vi "Calc min points to read.vi"(3 "error in":errorcluster, 4 "Target number of points":u64, 5 "Logging queue element":T1={"Imaging Protocol"=enum."Live Imaging", "Number of Trials"=0, "Frame Size"=512, "# Averaged frames"=0, "Dwell time (us)"=0.0, "Index of Z-plane"=0, "Timelapse?"=FALSE, "Logging process is active"=FALSE, "Speed logging enabled"=FALSE, "tdms file ref"=refnum, "path"=path "", "Trial Number"=0, "Expected # points acquired"=FALSE, "Manually stopped"=FALSE, "Last trial"=FALSE, "Ch0 data"=[], "Ch1 data"=[], "Image Time"=[], "Continuous Time"=[], "Points acquired"={"Ch0 last trial"=0, "Ch1 last trial"=0, "All trials"=0}, "HW Timings File"=refnum} {"Frame Size" items=["100X100"=100, "128X128"=128, "200X200"=200, "256X256"=256, "512X512"=512, "1024x1024"=1024, "2048x2048"=2048]; "Dwell time (us)" format="%#.6g"}) -> (0 "error out":errorcluster, 2 "Read at least # points":u32)   [LabVIEW 2017]
uses:
  Typedefs/Logging queue element.ctl
  Typedefs/Imaging Protocols enum.ctl
  Typedefs/Frame Size.ctl
  Typedefs/Acquired points count.ctl
panel:
  in  "Very important value":u64=200000
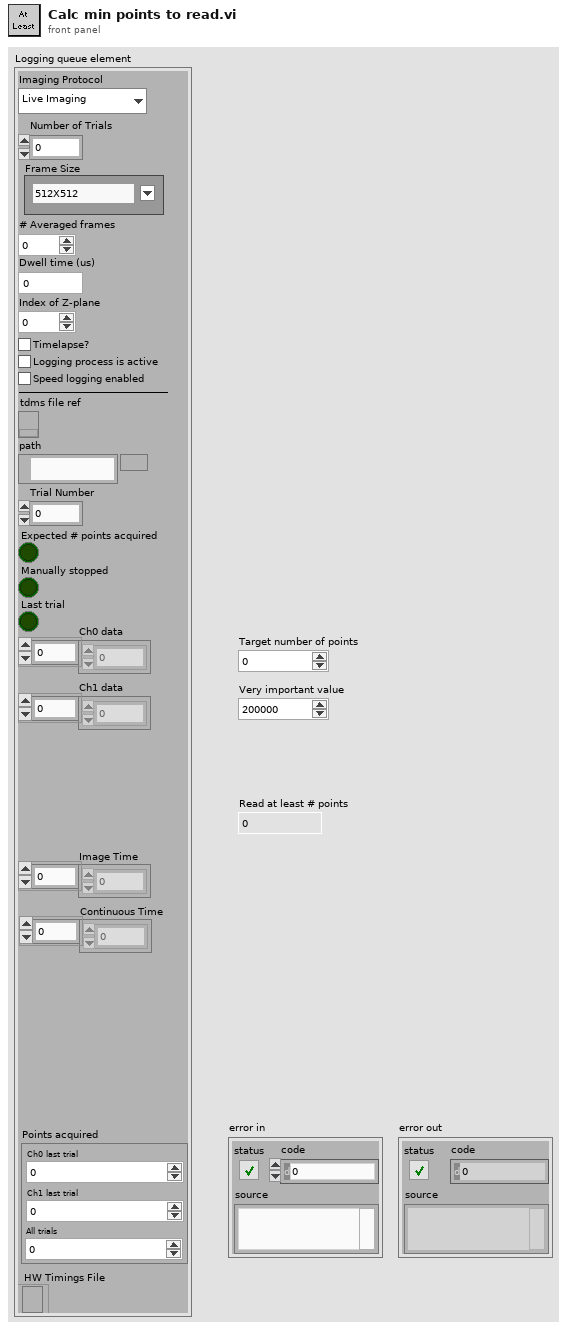
[diagram p1: front panel]
types:
  T1 = typedef "Logging queue element.ctl" = cluster{"Imaging Protocol":T2, "Number of Trials":u16, "Frame Size":T3, "# Averaged frames":u16, "Dwell time (us)":dbl, "Index of Z-plane":i32, "Timelapse?":bool, "Logging process is active":bool, "Speed logging enabled":bool, "tdms file ref":refnum<k34>, "path":path, "Trial Number":i32, "Expected # points acquired":bool, "Manually stopped":bool, "Last trial":bool, "Ch0 data":u32[], "Ch1 data":u32[], "Image Time":u64[], "Continuous Time":u64[], "Points acquired":T4, "HW Timings File":refnum<file>}
  T2 = typedef "Imaging Protocols enum.ctl" = enum16{"AOL Z-Stack", "Motor Z Stack", "Functional Acquisition", "Single Plane Acquisition", "Volume Acquisition", "Live Imaging", "Live Plane Imaging", "Live Volume Imaging"}
  T3 = typedef "Frame Size.ctl" = u16
  T4 = typedef "Acquired points count.ctl" = cluster{"Ch0 last trial":u64, "Ch1 last trial":u64, "All trials":u64}
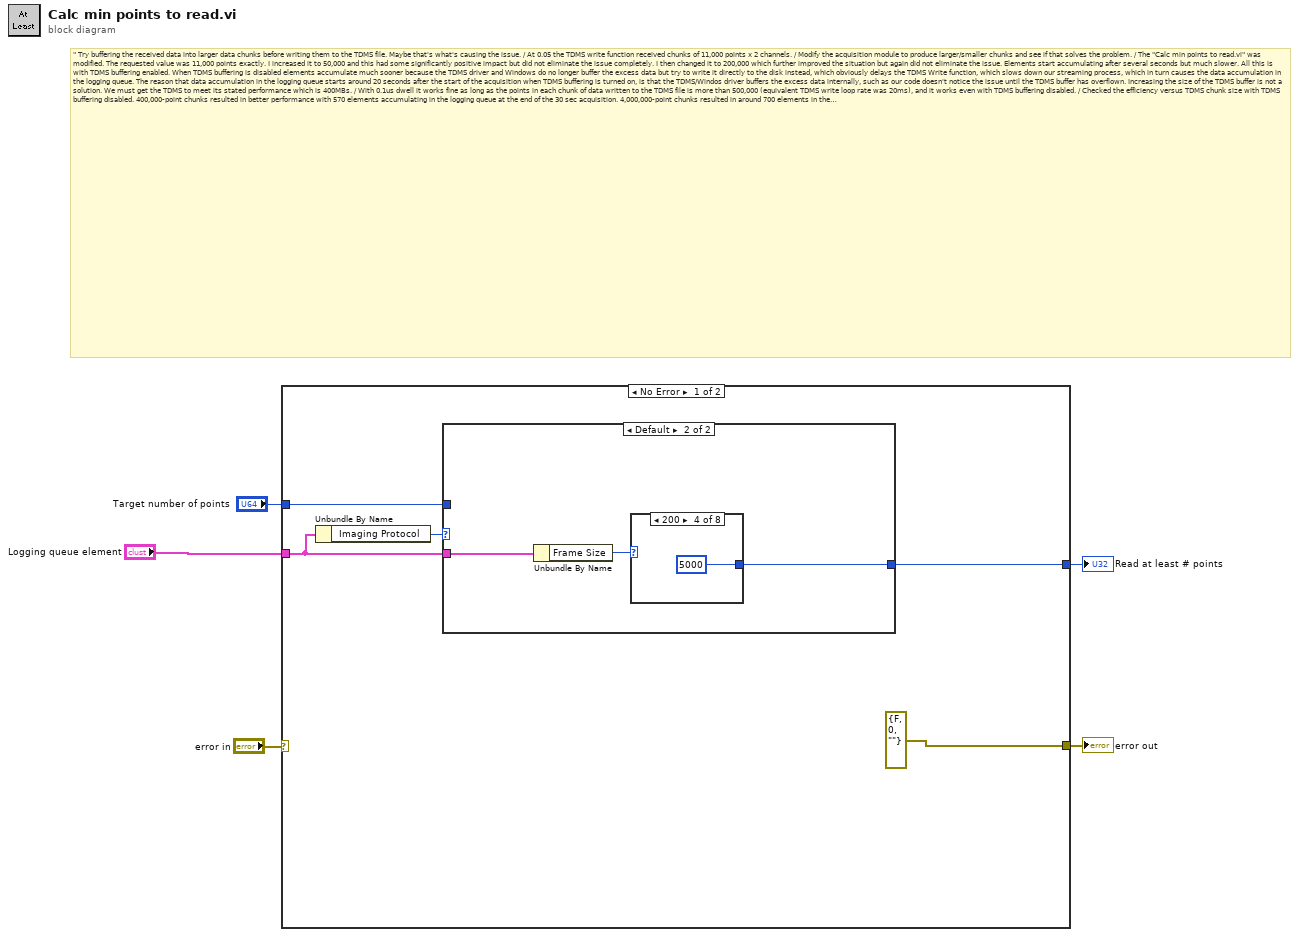
[diagram p0: block diagram]
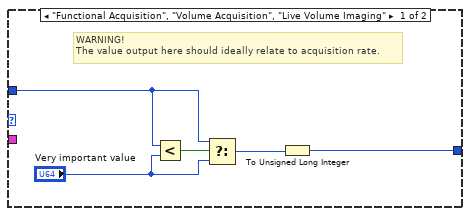
[diagram p2: hidden frame]
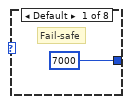
[diagram p3: hidden frame]
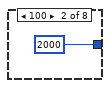
[diagram p4: hidden frame]
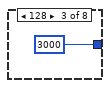
[diagram p5: hidden frame]
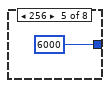
[diagram p6: hidden frame]
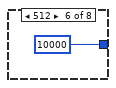
[diagram p7: hidden frame]
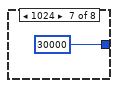
[diagram p8: hidden frame]
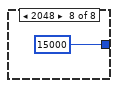
[diagram p9: hidden frame]
diagram:
  # "\"\tTry buffering the received data into larger data chunks before writing them to the TDMS file. Maybe that's what's causing the issue. / At 0.05 the TDMS write function received chunks of 11,000 points x 2 channels. / Modify the acquisition module to produce larger/smaller chunks and see if that solves the problem. / The \"Calc min points to read.vi\" was modified. The requested value was 11,000 points exactly. I increased it to 50,000 and this had some significantly positive impact but did not eliminate the issue completely. I then changed it to 200,000 which further improved the situation but again did not eliminate the issue. Elements start accumulating after several seconds but much slower. All this is with TDMS buffering enabled. When TDMS buffering is disabled elements accumulate much sooner because the TDMS driver and Windows do no longer buffer the excess data but try to write it directly to the disk instead, which obviously delays the TDMS Write function, which slows down our streaming process, which in turn causes the data accumulation in the logging queue. The reason that data accumulation in the logging queue starts around 20 seconds after the start of the acquisition when TDMS buffering is turned on, is that the TDMS/Windos driver buffers the excess data internally, such as our code doesn't notice the issue until the TDMS buffer has overflown. Increasing the size of the TDMS buffer is not a solution. We must get the TDMS to meet its stated performance which is 400MBs. / With 0.1us dwell it works fine as long as the points in each chunk of data written to the TDMS file is more than 500,000 (equivalent TDMS write loop rate was 20ms), and it works even with TDMS buffering disabled. / Checked the efficiency versus TDMS chunk size with TDMS buffering disabled. 400,000-point chunks resulted in better performance with 570 elements accumulating in the logging queue at the end of the 30 sec acquisition. 4,000,000-point chunks resulted in around 700 elements in the queue (note each element contained 4 Million points) as compared to the previous case where each element contained just 400,000 points). With 4,000-point chunks there were over 10,000 points in the queue before an error occurred. With 40,000-point chunks the queue size reached 3500 elements.\n4,000,000 -> 700 ' 2800M points in the queue\n400,000   -> 570 ' 228M points in the queue\n300,000  -> 600 ' 180M points\n200,000   -> 550  ' 110M points\n100,000   -> 2100 ' 210M points\n40,000    -> 3500 ' 140M points\n4,000      -> >10,000 ' N/A\nI set the chunk size to 200,000 points at least for now since it appears to be the most optimal value."
  n1 = case shown="No Error" "error in" {
    selector: "error in" -> [_ w27]
    tunnel: [w10 _] -> w5
    tunnel: "Logging queue element" -> [w6 _]
    tunnel: "Target number of points" -> [w8 _]
    tunnel: [errorcluster {"status"=FALSE, "code"=0, "source"=""} ("error out") w27] -> w3
    frame No Error {
      n2 = Unbundle By Name(w6) -> ("Imaging Protocol"=w9:T2)
      n3 = case shown="Default" w9 {
        tunnel: [w11 w18] -> w10
        tunnel: w6 -> [_ w16]
        tunnel: w8 -> [w14 _]
        frame "Functional Acquisition", "Volume Acquisition", "Live Volume Imaging" {
          # "WARNING!\nThe value output here should ideally relate to acquisition rate."
          n4 = Less?(x=w14, y="Very important value") -> (x < y?=w15:bool)
          n5 = Select(t=w14, s=w15, f="Very important value") -> (s? t:f=w12:u64)
          n6 = To Unsigned Long Integer(number=w12) -> (unsigned 32bit integer=w11:u32)
        }
        frame Default {
          n7 = Unbundle By Name(w16) -> ("Frame Size"=w17:T3)
          n8 = case shown="200" w17 {
            tunnel: [u32 7000 ("unsigned 32bit integer") u32 2000 ("unsigned 32bit integer") u32 3000 ("unsigned 32bit integer") u32 5000 ("unsigned 32bit integer") u32 6000 ("unsigned 32bit integer") u32 10000 ("unsigned 32bit integer") u32 30000 ("unsigned 32bit integer") u32 15000 ("unsigned 32bit integer")] -> w18
            frame Default {
              # "Fail-safe"
            }
            frame 100 {
            }
            frame 128 {
            }
            frame 200 {
            }
            frame 256 {
            }
            frame 512 {
            }
            frame 1024 {
            }
            frame 2048 {
            }
          }
        }
      }
    }
    frame Error {
    }
  }
  "Read at least # points" <- w5
  "error out" <- w3
